vi "Replace Control in VI (Array).vi"(8 "error in":errorcluster, 10 "Control Replacement Params":T1[](array[typedef])=[{"Placeholder Name"="PK", "CTL File Path"=path "C:/Users/OneEd/OneDrive/Desktop/MicroPort Job/CTDB/src/db_script/PK Test.ctl", "Indicator"=FALSE}, {"Placeholder Name"="Data", "CTL File Path"=path "C:/Users/OneEd/OneDrive/Desktop/MicroPort Job/CTDB/src/db_script/Value Test.ctl", "Indicator"=TRUE}], 11 "Original VI":path=path "C:/Users/OneEd/OneDrive/Desktop/MicroPort Job/CTDB/src/db_script/DB Select Template.vi") -> (0 "error out":errorcluster, 3 "Save as out":path=path "C:/Users/OneEd/OneDrive/Desktop/MicroPort Job/CTDB/src/db_script/DB Select Template.vi")   [LabVIEW 2022 SP3, in "EDT VI Script.lvlib"]
uses:
  EDT VI Script.lvlib
  Control Replacement Param.ctl
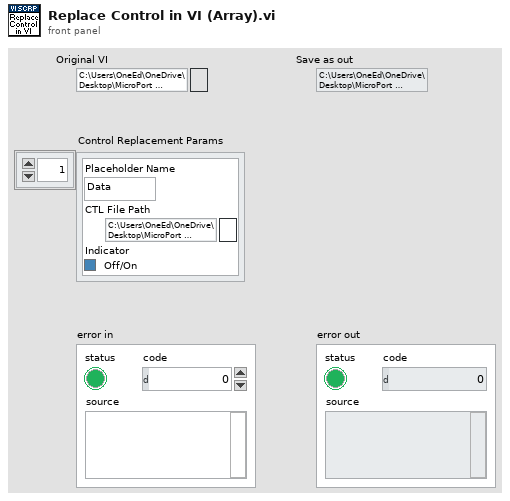
[diagram p1: front panel]
types:
  T1 = typedef "EDT VI Script.lvlib/Control Replacement Param.ctl" = cluster{"Placeholder Name":string, "CTL File Path":path, "Indicator":bool}
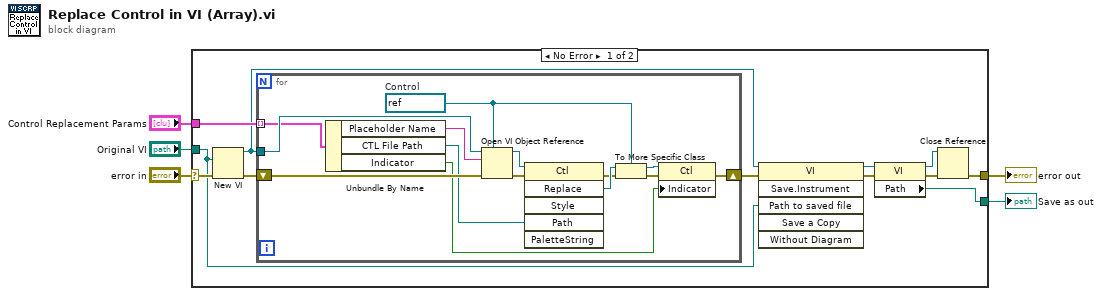
[diagram p0: block diagram]
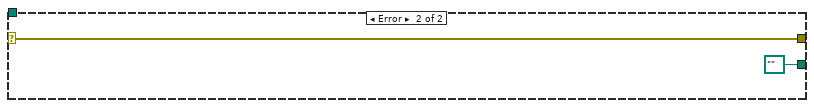
[diagram p2: hidden frame]
diagram:
  n1 = case shown="No Error" "error in" {
    selector: "error in" -> [w17 w33]
    tunnel: [w14 w33] -> w4
    tunnel: "Original VI" -> [w6 _]
    tunnel: "Control Replacement Params" -> [w15 _]
    tunnel: [w10 path "" ("Path")] -> w1
    frame No Error {
      n2 = New VI(8:w17, 10:w6) -> (0:w16:errorcluster, 3:w13:refnum<vi>)  [unwired: 5 in]
      n3 = for {
        tunnel: w13 -> [w31]
        shift-right: [w23] -> w9
        shift-left: w16 -> [w30]
        tunnel: w15 -> [w29] mode=indexing
        w21 = refnum<vi> refnum  # Control
        n4 = Unbundle By Name(w29) -> ("Placeholder Name"=w28:string, "CTL File Path"=w26:path, "Indicator"=w25:bool)
        n5 = Open VI Object Reference(7:w21, 8:w30, 10:w28, 11:w31) -> (0:w24:errorcluster, 3:w27:refnum<vi>)
        n6 = invoke on="Invoke Node" class="Ctl" method="Replace"(reference=w27, error in=w24, "Path"=w26) -> (error out=w19:errorcluster, "Replace"=w22:refnum<vi>)  [unwired: 3 in, 4 out]
        n7 = To More Specific Class(target class=w21, reference=w22, error in=w19) -> (specific class reference=w20:refnum<vi>, error out=w18:errorcluster)
        n8 = property class="Ctl"(reference=w20, error in=w18, "Indicator"=w25) -> (error out=w23:errorcluster)  [unwired: 1 out]
      }
      n9 = invoke class="VI" method="Save.Instrument"(reference=w13, error in=w9, "Path to saved file"=w6) -> (reference out=w8:refnum<vi>, error out=w7:errorcluster)  [unwired: 3 in, 4 out]
      n10 = property class="VI"(reference=w8, error in=w7) -> (reference out=w12:refnum<vi>, error out=w11:errorcluster, "Path"=w10:path)
      n11 = Close Reference(reference=w12, error in (no error)=w11) -> (error out=w14:errorcluster)
    }
    frame Error {
    }
  }
  "error out" <- w4
  "Save as out" <- w1
